vi "CameraQueryProperties.vi"(8 "error in (no error)":errorcluster, 11 "AndorSDK2 in":refnum<class "Andor2.lvclass">) -> (0 "error out":errorcluster, 1 "sensor_height":u16, 2 "sensor_width":u16, 3 "AndorSDK2 out":refnum<class "Andor2.lvclass">, 4 "cam_params":cluster{"String":string, "value":variant}[](array[cluster]) caption="params")   [LabVIEW 2010, in "Andor2.lvclass"]
uses:
  Andor2.lvclass
  Andor2.lvclass/Andor2.ctl
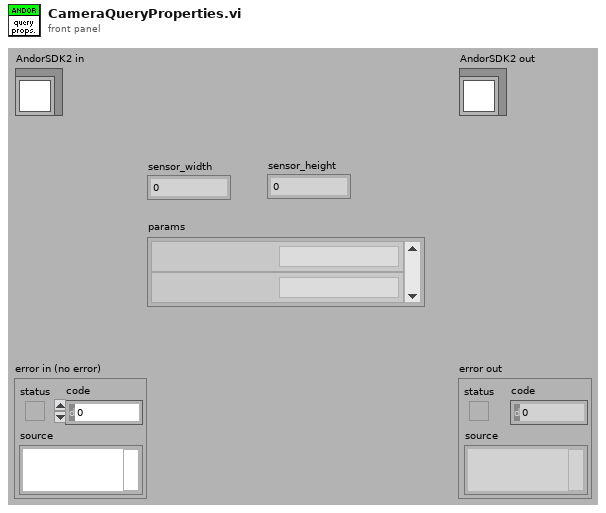
[diagram p1: front panel]
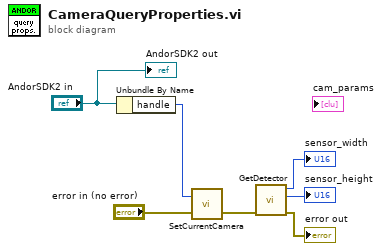
[diagram p0: block diagram]
diagram:
  n1 = Unbundle By Name("AndorSDK2 in") -> ("handle"=w2:i32)
  n2 = call <userlib>:"SetCurrentCamera.vi"("error in (no error)"="error in (no error)", "cameraHandle"=w2) -> ("error out"=w7:errorcluster)  [unwired: 1 out]
  n3 = call <userlib>:"GetDetector.vi"("error in (no error)"=w7) -> ("error out"=→"error out":errorcluster, "ypixels"=→"sensor_height":i32, "xpixels"=→"sensor_width":i32)  [unwired: 3 in, 1 out]
  "AndorSDK2 out" <- "AndorSDK2 in"
